vi "Progressbar_Update_Calib_frontpanel.vi"(7 "Ops":enum16{"Set Value", "Set Range"}(ring), 8 "error in (no error)":errorcluster, 9 "Value":dbl, 10 "Scale.Range:Minimum":dbl, 11 "Scale.Range:Maximum":dbl) -> (0 "error out":errorcluster)   [LabVIEW 2020]
uses:
  Globals/gl_Calibration globals.vi
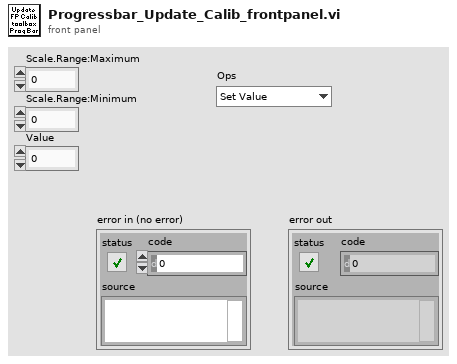
[diagram p1: front panel]
types:
  T1 = typedef "AOL Z cal process refs.ctl" = cluster{"This VI":refnum<vi>, "Abort (ind)":refnum<vi>, "Next (ind)":refnum<vi>, "Cancel":refnum<vi>, "Next":refnum<vi>, "Message":refnum<vi>, "Progress":refnum<vi>}
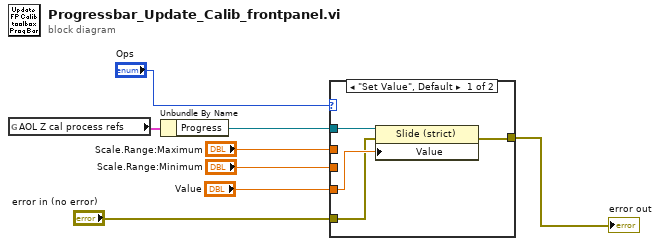
[diagram p0: block diagram]
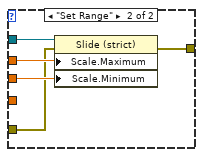
[diagram p2: hidden frame]
diagram:
  n1 = global read "gl_Calibration globals.vi" "AOL Z cal process refs"() -> (w7:T1)
  n2 = Unbundle By Name(w7) -> ("Progress"=w8:refnum<vi>)
  n3 = case shown="\"Set Value\", Default" "Ops" {
    tunnel: w8 -> [w12 w17]
    tunnel: "Scale.Range:Maximum" -> [_ w16]
    tunnel: "Scale.Range:Minimum" -> [_ w15]
    tunnel: "error in (no error)" -> [w10 w14]
    tunnel: [w9 w13] -> w3
    tunnel: "Value" -> [w11 _]
    frame "Set Value", Default {
      n4 = property class="Slide (strict)"(reference=w12, error in=w10, "Value"=w11) -> (error out=w9:errorcluster)  [unwired: 1 out]
    }
    frame "Set Range" {
      n5 = property class="Slide (strict)"(reference=w17, error in=w14, "Scale.Maximum"=w16, "Scale.Minimum"=w15) -> (error out=w13:errorcluster)  [unwired: 1 out]
    }
  }
  "error out" <- w3
